vi "test-PLT.vi"() -> ()   [LabVIEW 2014]
doc: "André Romero - 2016\nandretec@ifsc.usp.br"
panel:
  out "Rotation (deg)":dbl=54.0
  in  "Scale by":enum16{"X", "Y", "XY"}(ring)=enum."Y"
  in  "offset Y":dbl format="%0.2f"
  in  "Scale":dbl=5.0
  in  "offset X":dbl format="%0.2f"
  out "XY Graph":cluster{"Y":dbl[], "Y":dbl[]}(graph)={"Y"=[-7.2103015218218545, -8.32188065086848, -9.26992047514052, -6.223757436618837, 0.5820141516292439, 0.560280250146286, 0.6312931651534024, 0.6025697878464462, 0.4899727006515042, 0.28861648524527084, -2.7779158011381204, -3.0969749487852036, -3.4983628272031444, -3.9531797177069015, -4.1891005752276484, -4.4150742547237005, -4.7962291254312905, -5.172925400165578, -5.893430542670331, -7.398287925484872, -8.272473365428556, -8.70808723430005, -6.223757436618837, -3.693521110927855, -1.4522740038516726, 3.105812024961281, 3.678552274428494, 4.357120561989254, 5.522244936001151, 5.8067093872844096, 5.927075455409518, 5.886344927921694, 5.679029222769549, 3.071081088446093, 2.639424853604067, 2.1783098216934373, 1.7659447791727163, 1.3744599934349497, 0.9864479029369217, 0.5820141516292439, -1.0151632253253677, -0.6950380611741864, -1.0920114289633438, -1.488513889057979, -1.8735241920107901, -2.2454973587046476, -2.890046051439251, -3.8924567031861526, -5.629072905923472, -5.801485317300144, -5.902031168969698, -5.903311636019701, -5.780929681082942, -5.572319477785586, -5.286398218074241, -4.684155086193903, -4.084398748819739, -3.784542622804917, -3.4418078264570586, 0.9950584895307832, 3.3418691226333883, 9.099391694541936, 0.43363803994510874, -0.6950380611741864, -0.6607820164713201, -0.7467156985154766, -0.7798676175464241, -0.6842953548892172, -0.48246823178846254, -0.2023441515401534, 2.417567047619648, 2.797898327876551, 3.207688405202057, 3.4440360850728045, 3.702853086188157, 4.000605154702285, 4.334805496109016, 4.85012904521163, 5.334581074162075, 6.274629498722445, 11.702837147547566, 10.503572961712258, 9.099391694541936, 6.722729480387837], "Y"=[-1.4407047190276656, -2.9475779886538565, -4.321695302968591, -6.534862297692626, -6.1126282008588415, -6.558056991721468, -6.945083181485931, -7.377048013739603, -7.647445342685821, -7.9707566906788125, -12.191476288198043, -12.538286943513725, -12.825282274647677, -12.989601084528429, -13.002682306131906, -12.955904118209126, -12.78799438815028, -12.556237560286398, -12.024374125435777, -10.956188659761233, -10.312669953104717, -9.954248915708856, -6.534862297692626, -8.373186594211148, 1.6714956534298855, 2.3934255580545134, 2.1198641312802025, 1.6687844480833092, 0.7216423538557928, 0.3975655318518405, 0.06692605637389004, -0.2892286132384019, -0.6669107887062546, -4.2564434503155875, -4.8736514345774875, -5.427527314073398, -5.706547268649786, -5.841407281461935, -5.936861319180785, -6.1126282008588415, -4.9522109117332676, 5.69159644736343, 5.560724122830062, 5.488210314050338, 5.373803735671142, 5.115752208566752, 4.309401554706882, 2.9412437301380594, 0.5048282923597571, 0.15210223264268352, -0.28638116774046507, -0.7382844413880476, -1.112317580238078, -1.3561256436273461, -1.5974028271659202, -2.0265722675017726, -2.4707065602191878, -2.64663575218012, -2.7866316642874933, -2.0353311332833033, 8.385488310708453, 4.20240330626609, 4.821250416510858, 5.69159644736343, 6.027297682542769, 6.324534758017855, 6.8098404316683006, 7.218394127288324, 7.600063991034959, 8.008705857344022, 11.614704265107527, 12.126643289659444, 12.575250209445372, 12.738965855598039, 12.852813355593671, 12.904829644595921, 12.880049870223228, 12.723676382650725, 12.455559452583282, 11.76418848658138, 7.82036477886594, 6.100466795313608, 4.20240330626609, 0.9312084036374007]}
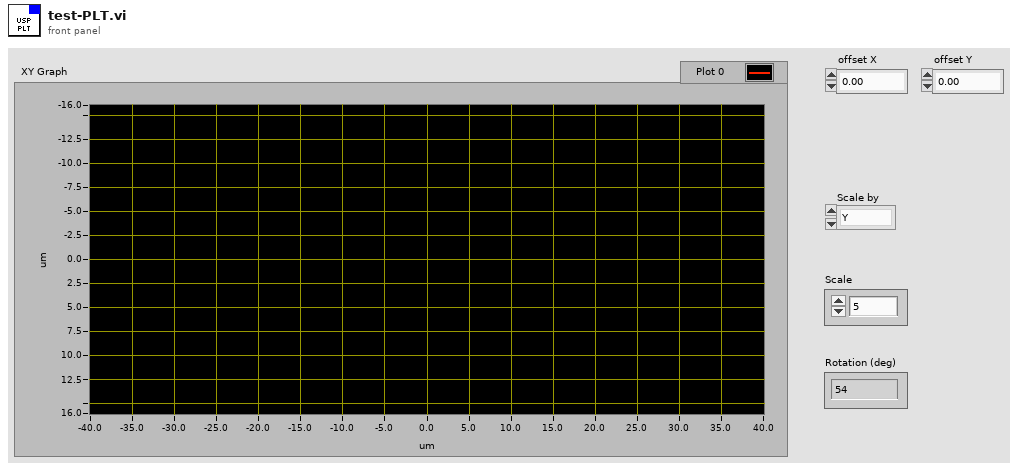
[diagram p1: front panel]
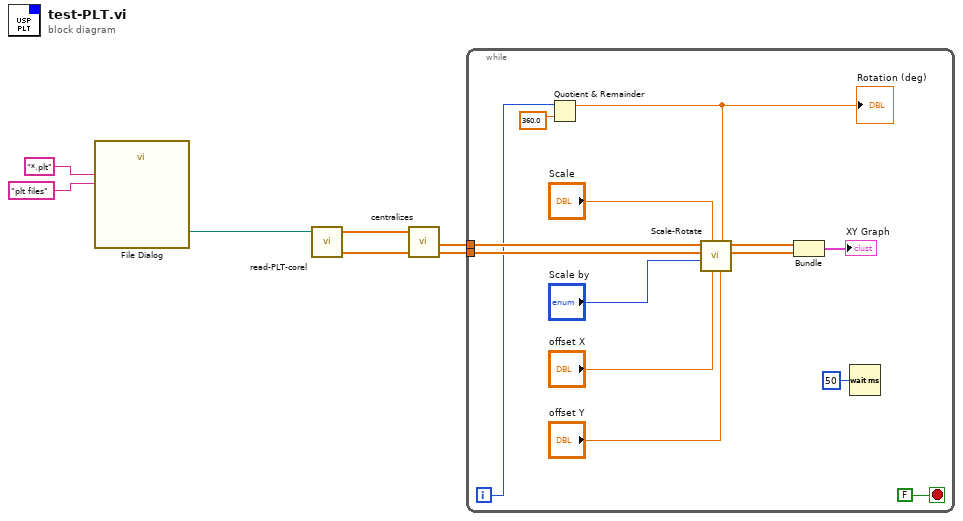
[diagram p0: block diagram]
diagram:
  n1 = call "File Dialog"("pattern (all files)"="*.plt", "pattern label"="plt files") -> ("selected path"=w3:path)  [unwired: 10 in, 3 out]
  n2 = call "read-PLT-corel.vi"("file (use dialog)"=w3) -> ("Y"=w5:ext[], "X"=w7:ext[])  [unwired: 2 in, 1 out]
  n3 = call "centralizes.vi"("Y in"=w5, "X in"=w7) -> ("Y out"=w4:ext[], "X out"=w6:ext[])  [unwired: 2 in]
  n4 = while {
    tunnel: w6 -> [w17]
    tunnel: w4 -> [w16]
    i -> [w11]
    stop <- FALSE stop-if-true
    n5 = Quotient & Remainder(x=w11, y=360.0) -> (x-y*floor(x/y)=w10:dbl)  [unwired: 1 out]
    "Rotation (deg)" <- w10
    n6 = call "Scale-Rotate.vi"("offset Y"="offset Y", "Rotation (deg)"=w10, "offset X"="offset X", "Scale"="Scale", "Scale by"="Scale by", "Y in"=w16, "X in"=w17) -> ("Y out"=w14:dbl[], "X out"=w15:dbl[])  [unwired: 3 in]
    n7 = Bundle("X out"=w15, "Y out"=w14) -> (→"XY Graph":cluster{"X out":dbl[], "Y out":dbl[]})  [unwired: 1 in]
    n8 = Wait (ms)(milliseconds to wait=u32 50) -> ()  [unwired: 1 out]
  }
